vi "Calculate G.vi"(8 "Frequency (fihat)":dbl, 9 "Subharmonic (h)":dbl, 10 "Center frequency of bin (b)":dbl) -> (2 "G":dbl)   [LabVIEW 2014]
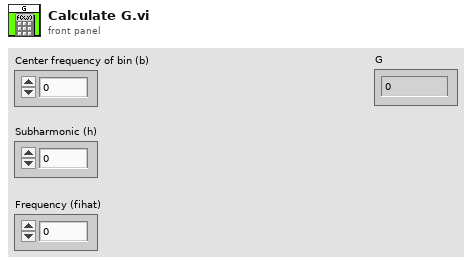
[diagram p1: front panel]
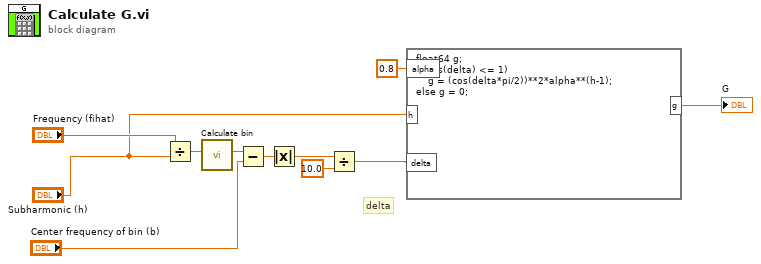
[diagram p0: block diagram]
diagram:
  # "delta"
  n1 = Divide(x="Frequency (fihat)", y="Subharmonic (h)") -> (x/y=w10:dbl)
  n2 = call "Calculate bin.vi"("Frequency"=w10) -> ("B"=w9:dbl)  [unwired: 10 in]
  n3 = Subtract(x=w9, y="Center frequency of bin (b)") -> (x-y=w7:dbl)
  n4 = Absolute Value(x=w7) -> (abs(x)=w6:dbl)
  n5 = Divide(x=w6, y=10.0) -> (x/y=w4:dbl)
  n6 = formula code="float64 g;\nif(abs(delta) <= 1)\n    g = (cos(delta*pi/2))**2*alpha**(h-1);\nelse g = 0;"("delta"=w4, "alpha"=0.8 ("input variable"), "h"="Subharmonic (h)") -> ("g"=→"G":dbl)
